vi "CTR_ReadXML_Config.vi"(8 "error in":errorcluster, 10 "StreamCluster_TypeDef":T1={"DAQ_Configs"=[], "CTR_Config"={"CTR refDes"="", "CTR IP Addr"=""}, "Network_Configs"={"Buffer"=1, "ManagmentRate_Hz"=1000, "StreamRate_Hz"=10, "ConnectionHysterisis"=0, "LoggingRate_Hz"=10}, "ConfigXML_Checksum"=""}, 11 "path":path) -> (0 "error out":errorcluster={"status"=TRUE, "code"=0, "source"=""}, 2 "StreamCluster_TypeDef out":T1={"DAQ_Configs"=[], "CTR_Config"={"CTR refDes"="", "CTR IP Addr"="localhost"}, "Network_Configs"={"Buffer"=1, "ManagmentRate_Hz"=1000, "StreamRate_Hz"=10, "ConnectionHysterisis"=0, "LoggingRate_Hz"=10}, "ConfigXML_Checksum"="210cc09a95e8171523621a6e0fe6cc62ee78011ce952e85bacd084a90afd4457596a89e2a0760488e968f21beda495caaa4ef384b0090342ba5af4eb26a7085d"})   [LabVIEW 2024]
uses:
  Control/StreamCluster_TypeDef.ctl
  Control/streamIO_states.ctl
  <vilib>/security/Message Digest/API/Instances/File/SHA3-512 File Checksum.vi
  <vilib>/xml/Close Reference(Node).vi
  <vilib>/xml/Load XML File.vi
  <vilib>/xml/NI_XML.lvlib
  <vilib>/security/Message Digest/API/NI_Message Digest API.lvlib
panel:
  out "Input Array":string[][][](array[string])
  out "Control Array":string[][][](array[string])
  out "parse errors":string
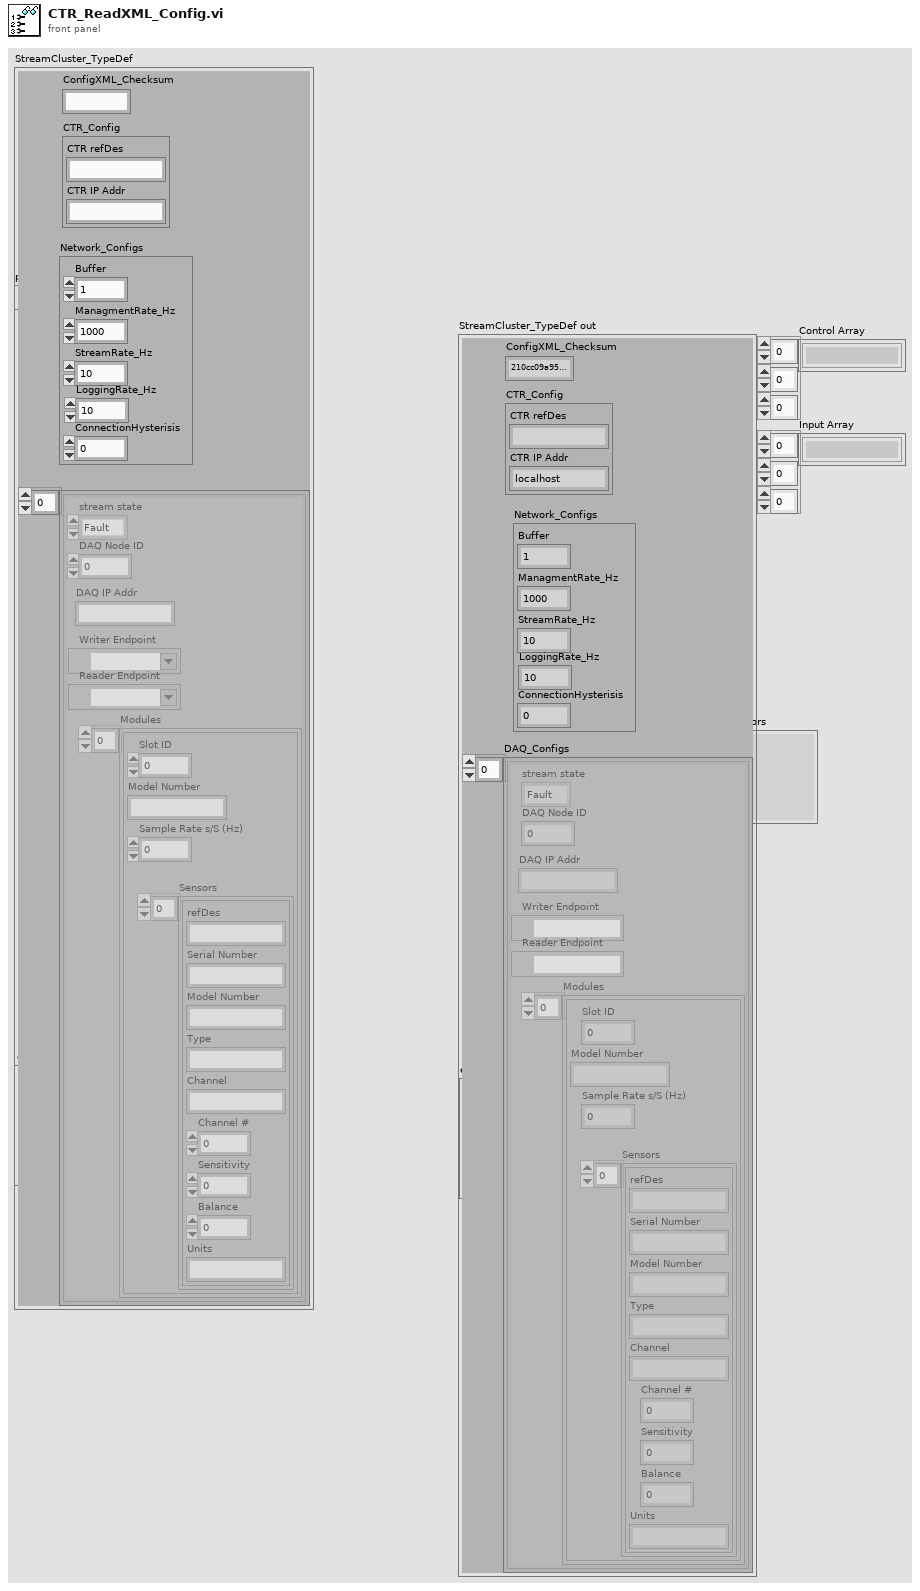
[diagram p1: front panel]
types:
  T1 = typedef "StreamCluster_TypeDef.ctl" = cluster{"DAQ_Configs":cluster{"stream state":T2, "DAQ Node ID":i32, "Writer Endpoint":refnum<k21>, "Reader Endpoint":refnum<k21>, "Modules":cluster{"Slot ID":i32, "Model Number":string, "Sample Rate s/S (Hz)":dbl, "Sensors":cluster{"refDes":string, "Serial Number":string, "Model Number":string, "Type":string, "Channel":string, "Channel #":i32, "Sensitivity":dbl, "Balance":dbl, "Units":string}[]}[], "DAQ IP Addr":string}[], "CTR_Config":cluster{"CTR refDes":string, "CTR IP Addr":string}, "Network_Configs":cluster{"Buffer":i32, "ManagmentRate_Hz":i32, "StreamRate_Hz":i32, "ConnectionHysterisis":i32, "LoggingRate_Hz":i32}, "ConfigXML_Checksum":string}
  T2 = typedef "streamIO_states.ctl" = enum16{"Fault", "Initialize", "Stream", "Close"}
  T3 = cluster{"stream state":T2, "DAQ Node ID":i32, "Writer Endpoint":refnum<k21>, "Reader Endpoint":refnum<k21>, "Modules":cluster{"Slot ID":i32, "Model Number":string, "Sample Rate s/S (Hz)":dbl, "Sensors":cluster{"refDes":string, "Serial Number":string, "Model Number":string, "Type":string, "Channel":string, "Channel #":i32, "Sensitivity":dbl, "Balance":dbl, "Units":string}[]}[], "DAQ IP Addr":string}[]
  T4 = cluster{"Slot ID":i32, "Model Number":string, "Sample Rate s/S (Hz)":dbl, "Sensors":cluster{"refDes":string, "Serial Number":string, "Model Number":string, "Type":string, "Channel":string, "Channel #":i32, "Sensitivity":dbl, "Balance":dbl, "Units":string}[]}[]
  T5 = cluster{"refDes":string, "Serial Number":string, "Model Number":string, "Type":string, "Channel":string, "Channel #":i32, "Sensitivity":dbl, "Balance":dbl, "Units":string}[]
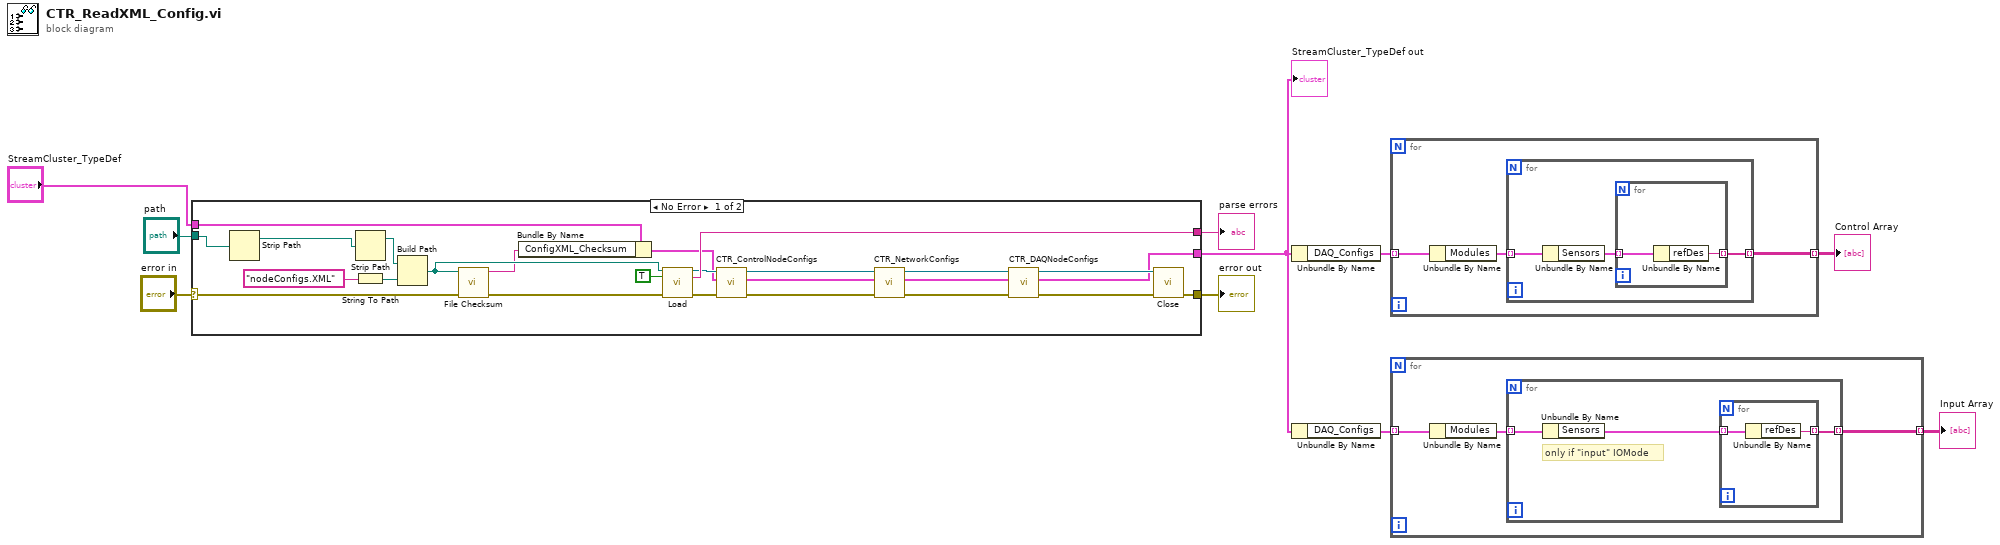
[diagram p0: block diagram]
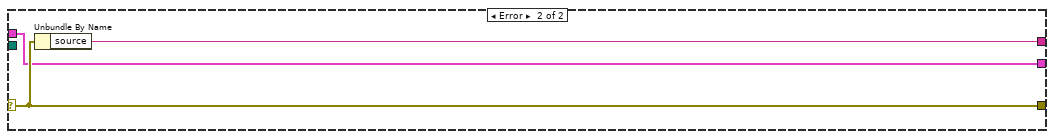
[diagram p2: hidden frame]
diagram:
  n1 = case shown="No Error" "error in" {
    selector: "error in" -> [w34 w38]
    tunnel: [w25 w38] -> w7
    tunnel: "path" -> [w30 _]
    tunnel: "StreamCluster_TypeDef" -> [w20 w36]
    tunnel: [w26 w37] -> w8
    tunnel: [w11 w36] -> w1
    frame No Error {
      n2 = Strip Path(path=w30) -> (stripped path=w29:path)  [unwired: 1 out]
      n3 = String To Path(string="nodeConfigs.XML") -> (path=w32:path)
      n4 = Strip Path(path=w29) -> (stripped path=w28:path)  [unwired: 1 out]
      n5 = Build Path(base path=w28, name or relative path=w32) -> (appended path=w35:path)
      n6 = call-poly <vilib>:"File Checksum.vi"("error in"=w34, "path"=w35) -> ("error out"=w33:errorcluster, "digest"=w18:string)  [unwired: 8 in]
      n7 = Bundle By Name(cluster=w20, "ConfigXML_Checksum"=w18) -> (w19:T1)
      n8 = call-poly <vilib>:"Load.vi"("path to XML document"=w35, "process namespaces (False)"=TRUE, "error in (no error)"=w33) -> ("DOM document out"=w22:refnum<k20>, "parse errors"=w26:string, "error out"=w21:errorcluster)  [unwired: 10 in]
      n9 = call "CTR_ControlNodeConfigs.vi"("error in"=w21, "StreamCluster_TypeDef in"=w19, "DOM document in"=w22) -> ("error out"=w23:errorcluster, "StreamCluster_TypeDef out"=w17:T1, "DOM document out"=w24:refnum<k20>)  [unwired: 6 in]
      n10 = call "CTR_NetworkConfigs.vi"("error in"=w23, "StreamCluster_TypeDef"=w17, "DOM document in"=w24) -> ("error out"=w16:errorcluster, "StreamCluster_TypeDef 2"=w15:T1, "DOM document out"=w14:refnum<k20>)  [unwired: 6 in]
      n11 = call "CTR_DAQNodeConfigs.vi"("error in"=w16, "StreamCluster_TypeDef in"=w15, "DOM document in"=w14) -> ("error out"=w13:errorcluster, "StreamCluster_TypeDef out"=w11:T1, "DOM document out"=w12:refnum<k20>)  [unwired: 6 in]
      n12 = call-poly <vilib>:"Close.vi"("error in (no error)"=w13, "node"=w12) -> ("error out"=w25:errorcluster)  [unwired: 7 in]
    }
    frame Error {
      n13 = Unbundle By Name(w38) -> ("source"=w37:string)
    }
  }
  "error out" <- w7
  "parse errors" <- w8
  "StreamCluster_TypeDef out" <- w1
  n14 = Unbundle By Name(w1) -> ("DAQ_Configs"=w5:T3)
  n15 = Unbundle By Name(w1) -> ("DAQ_Configs"=w2:T3)
  n16 = for {
    tunnel: w5 -> [w41] mode=indexing
    tunnel: [w39] -> w4 mode=indexing
    n17 = Unbundle By Name(w41) -> ("Modules"=w40:T4)
    n18 = for {
      tunnel: w40 -> [w44] mode=indexing
      tunnel: [w42] -> w39 mode=indexing
      n19 = Unbundle By Name(w44) -> ("Sensors"=w43:T5)
      n20 = for {
        tunnel: w43 -> [w46] mode=indexing
        tunnel: [w45] -> w42 mode=indexing
        n21 = Unbundle By Name(w46) -> ("refDes"=w45:string)
      }
    }
  }
  "Control Array" <- w4
  n22 = for {
    tunnel: w2 -> [w49] mode=indexing
    tunnel: [w47] -> w3 mode=indexing
    n23 = Unbundle By Name(w49) -> ("Modules"=w48:T4)
    n24 = for {
      tunnel: w48 -> [w52] mode=indexing
      tunnel: [w50] -> w47 mode=indexing
      # "only if \"input\" IOMode"
      n25 = Unbundle By Name(w52) -> ("Sensors"=w51:T5)
      n26 = for {
        tunnel: w51 -> [w54] mode=indexing
        tunnel: [w53] -> w50 mode=indexing
        n27 = Unbundle By Name(w54) -> ("refDes"=w53:string)
      }
    }
  }
  "Input Array" <- w3
